vi "Remove From Child List.vi"(8 "error in (no error)":errorcluster, 10 "Child ID":string, 11 "Generic Node in":refnum<class "Generic Node.lvclass">) -> (0 "error out":errorcluster, 3 "Generic Node out":refnum<class "Generic Node.lvclass">)   [LabVIEW 2017, in "opcua.lvlib" / "Browser Core.lvlib" / "Generic Node.lvclass"]
doc: "Remove UID from Child List"
uses:
  Generic Node.lvclass
  Generic Node.lvclass/Generic Node.ctl
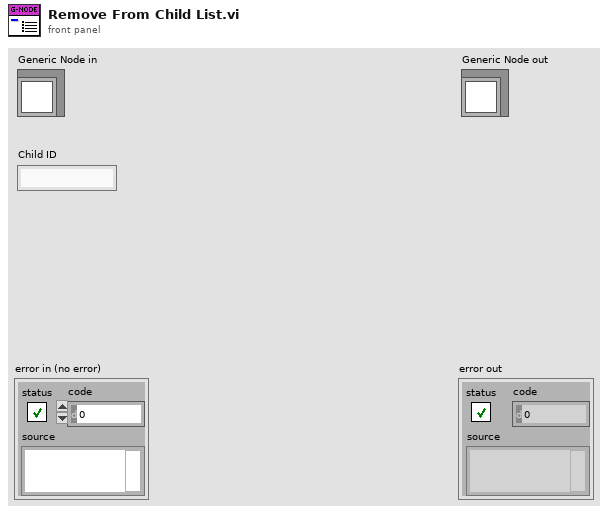
[diagram p1: front panel]
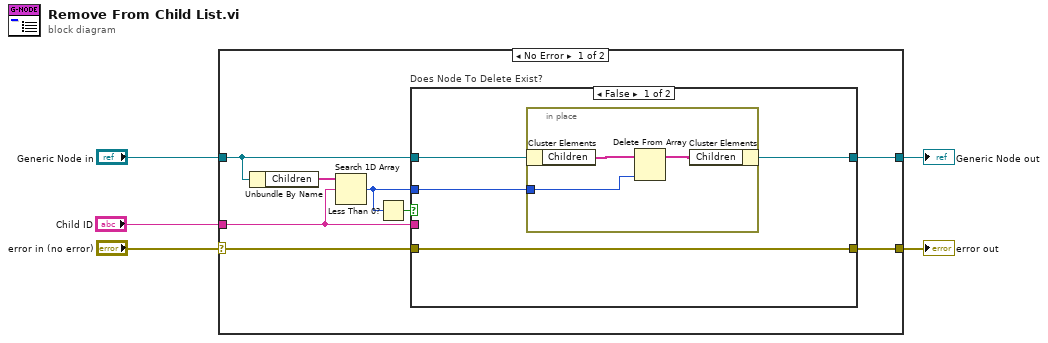
[diagram p0: block diagram]
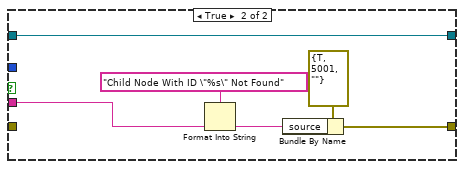
[diagram p2: hidden frame]
diagram:
  n1 = case shown="No Error" "error in (no error)" {
    selector: "error in (no error)" -> [w10 w28]
    tunnel: [w9 w28] -> w4
    tunnel: [w6 w27] -> w2
    tunnel: "Generic Node in" -> [w11 w27]
    tunnel: "Child ID" -> [w8 _]
    frame No Error {
      n2 = Unbundle By Name(w11) -> ("Children"=w13:string[])
      n3 = Search 1D Array(1D array=w13, element=w8) -> (index of element=w7:i32)  [unwired: 1 in]
      n4 = Less Than 0?(x=w7) -> (x < 0?=w12:bool)
      n5 = case "Does Node To Delete Exist?" shown="False" w12 {
        tunnel: w11 -> [w17 w21]
        tunnel: w10 -> [w14 _]
        tunnel: [w14 w22] -> w9
        tunnel: w8 -> [_ w23]
        tunnel: w7 -> [w16 _]
        tunnel: [w15 w21] -> w6
        frame False {
          n6 = in-place {
            in-place-border: w16 -> [w19]
            n7 = in-place-cluster #1(w17) -> ("Children"=w20:string[])
            n8 = Delete From Array(array=w20, index=w19) -> (array with subset deleted=w18:string[])  [unwired: 1 in, 1 out]
            n9 = in-place-cluster #1("Children"=w18) -> (w15:refnum<class "Generic Node.lvclass">)
          }
        }
        frame True {
          n10 = Format Into String(format string="Child Node With ID \"%s\" Not Found", w23) -> (resulting string=w24:string)  [unwired: 2 in, 1 out]
          n11 = Bundle By Name(cluster=errorcluster {"status"=TRUE, "code"=5001, "source"=""} ("error IO"), "source"=w24) -> (w22:errorcluster)
        }
      }
    }
    frame Error {
      # "Do Not Edit Child List on Error In"
    }
  }
  "error out" <- w4
  "Generic Node out" <- w2
